vi "addToImagePathQ.vi"(8 "error in (no error)":errorcluster, 10 "ImagePath":path, 11 "ImageStreamDecoder in":refnum<class "ImageStreamDecoder.lvclass">) -> (0 "error out":errorcluster, 3 "ImageStreamDecoder out":refnum<class "ImageStreamDecoder.lvclass">)   [LabVIEW 2011, in "Hardware.lvlib" / "HWControllers.lvlib" / "ImageStreamDecoder.lvclass"]
uses:
  ImageStreamDecoder.lvclass
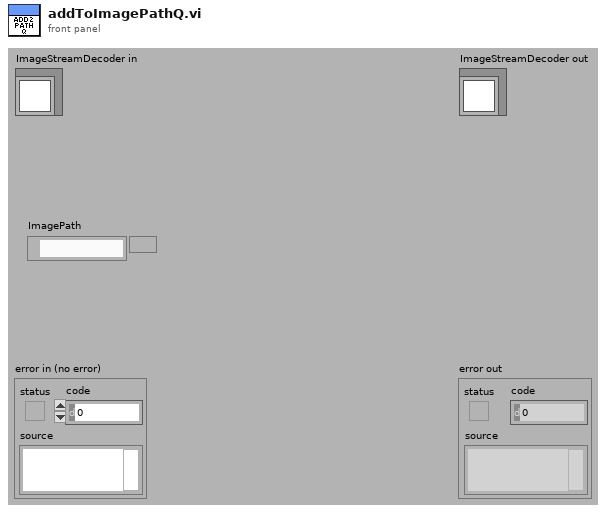
[diagram p1: front panel]
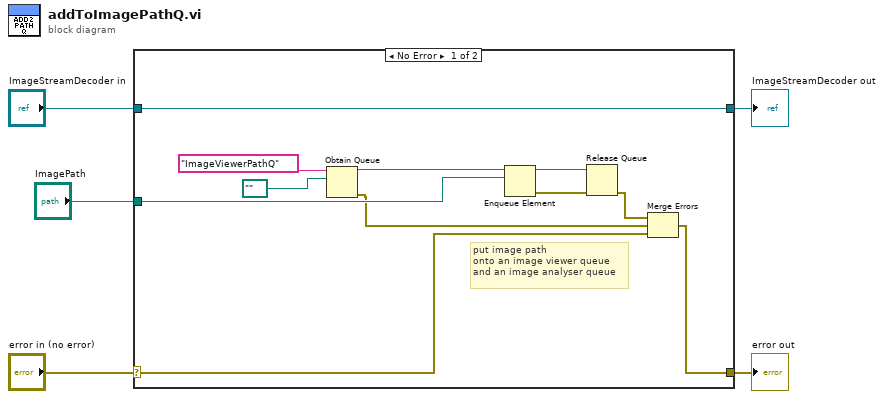
[diagram p0: block diagram]
diagram:
  n1 = case shown="No Error" "error in (no error)" {
    selector: "error in (no error)" -> [w7 w18]
    tunnel: [w6 w18] -> w4
    tunnel: [w16 w17] -> w2
    tunnel: "ImageStreamDecoder in" -> [w16 w17]
    tunnel: "ImagePath" -> [w10 _]
    frame No Error {
      # "put image path\nonto an image viewer queue\nand an image analyser queue"
      n2 = Obtain Queue(name (unnamed)="ImageViewerPathQ", element data type=path "") -> (queue out=w13:refnum<queue>, error out=w8:errorcluster)  [unwired: 3 in, 1 out]
      n3 = Enqueue Element(queue=w13, element=w10) -> (queue out=w11:refnum<queue>, error out=w12:errorcluster)  [unwired: 2 in, 1 out]
      n4 = Release Queue(queue=w11, error in (no error)=w12) -> (error out=w9:errorcluster)  [unwired: 1 in, 2 out]
      n5 = Merge Errors(w9, w8, w7) -> (w6:errorcluster)
    }
    frame Error {
    }
  }
  "error out" <- w4
  "ImageStreamDecoder out" <- w2
